vi "Watchdog Simple.vi"() -> ()   [LabVIEW 2021]
panel:
  out "Address Found":string
  out "Device Type Found":string
  in  "Enable Watchdog w/ Reset":bool
  in  "Timeout [s]":i32=10 min=1 max=50
  out "Error Message":string
  out "error out":errorcluster
  # "Simple example opens the first found device and enables the watchdog\nto reset the device after the specified timeout.  This example does not disable\nthe watchdog, but rather just enables/disables the reset option of the watchdog."
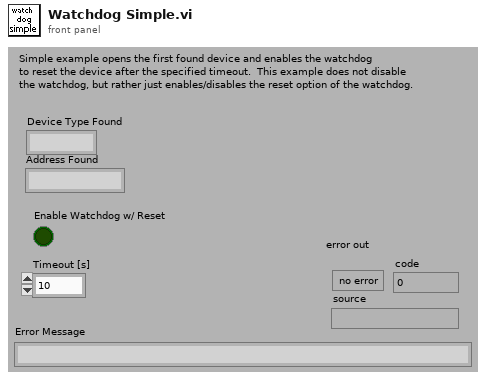
[diagram p1: front panel]
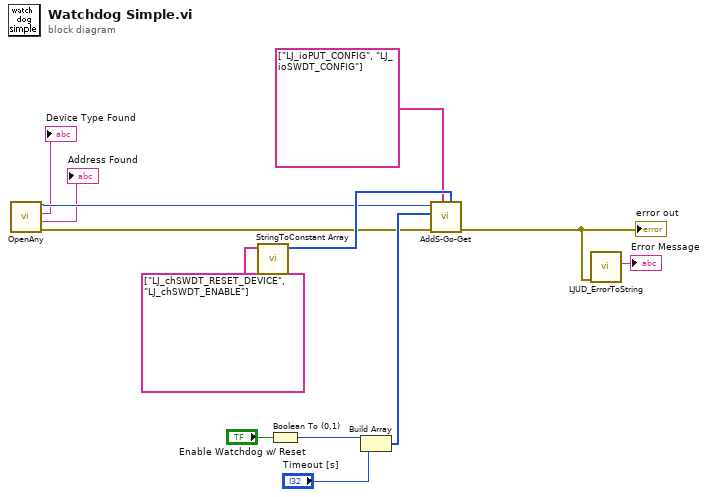
[diagram p0: block diagram]
diagram:
  n1 = call "OpenAny.vi"() -> ("error out"=w4:errorcluster, "Address Found"=→"Address Found":string, "Device Type Found"=→"Device Type Found":string, "Handle"=w3:i32)  [unwired: 8 in]
  n2 = call "StringToConstant Array.vi"("String Constant Array In"=string[] ["LJ_chSWDT_RESET_DEVICE", "LJ_chSWDT_ENABLE"] ("IOTypes")) -> ("I32 Constant Array Out"=w11:i32[])  [unwired: 10 in]
  n3 = Boolean To (0,1)(Boolean="Enable Watchdog w/ Reset") -> (0, 1=w6:i16)
  n4 = Build Array(w6, "Timeout [s]") -> (w5:i32[])
  n5 = call "AddS-Go-Get.vi"("Channels"=w11, "IOTypes"=string[] ["LJ_ioPUT_CONFIG", "LJ_ioSWDT_CONFIG"], "error in"=w4, "Values Write"=w5, "Handle In"=w3) -> ("error out"=w9:errorcluster)  [unwired: 4 in, 2 out]
  "error out" <- w9
  n6 = call "LJUD_ErrorToString.vi"("error in"=w9) -> ("String"=→"Error Message":string)  [unwired: 10 in]
